vi "GSI-HVSwitch2.get revision.vi"(0 "i ref in":refnum<vi>, 3 "ms timeout (10000)":i32=10000, 5 "error in (no error)":errorcluster) -> (14 "i ref out":refnum<vi>, 15 "revisionType":T1, 16 "revision":string, 17 "timed out":bool, 19 "error out":errorcluster)   [LabVIEW 2014, in "GSI-HVSwitch2.lvlib"]
doc: "Queries the revision number from the device."
uses:
  GSI-HVSwitch2.lvlib
  CSinstr.lib/SDEX/SDEX.revisionType.ctl
  CSCore/CSApplicationBaseClasses/DeviceBase/DeviceBase.lvlib
  CSlibraries-extern/DimLVEvent/NodeMon-LV/LVNodeInfo/LVNodeInfo.lvlib
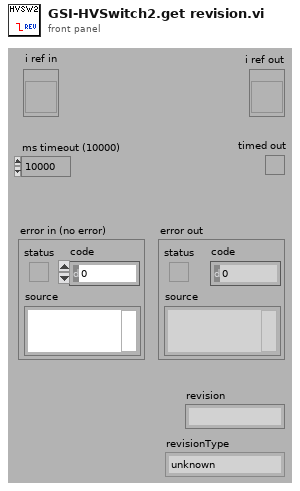
[diagram p1: front panel]
types:
  T1 = typedef "SDEXDriver.lvlib/SDEX.revisionType.ctl" = enum16{"unknown", "hvamp3", "hvswi1", "htrp0", "WDG0"}
  T2 = typedef "GSI-HVSwitch2.lvlib/GSI-HVSwitch2.i attribute.ctl" = cluster{"SDEX VISA Cluster":T3, "SetVoltage SW0":dbl, "SetVoltage SW1":dbl, "ActTempAmp":dbl, "ActTempPS1":dbl, "ActTempPS2":dbl, "mode":T5, "interfaceInitialized":bool, "serviceIDs":cluster{"nomVoltage0ID":i32, "nomVoltage1ID":i32, "actTempAmpID":i32, "actTempPS1ID":i32, "actTempPS2ID":i32, "modeID":i32}, "usedChannels":i32}
  T3 = typedef "SDEXDriver.lvlib/SDEX.VISA Control.ctl" = cluster{"VISA resource name":refnum<visa-resource-name>, "HEX address":u16, "VISA Timeout Value (1000 ms)":u32, "Lock Timeout (1000 ms)":u32, "semaphore":T4, "Baud rate":u32, "revision":T1, "deviceInfo":string}
  T4 = typedef "Semaphore RefNum" = refnum<k1>
  T5 = typedef "GSI-HVSwitch2.lvlib/GSI-HVSwitch2.mode.ctl" = enum16{"unknown", "switch", "stepper"}
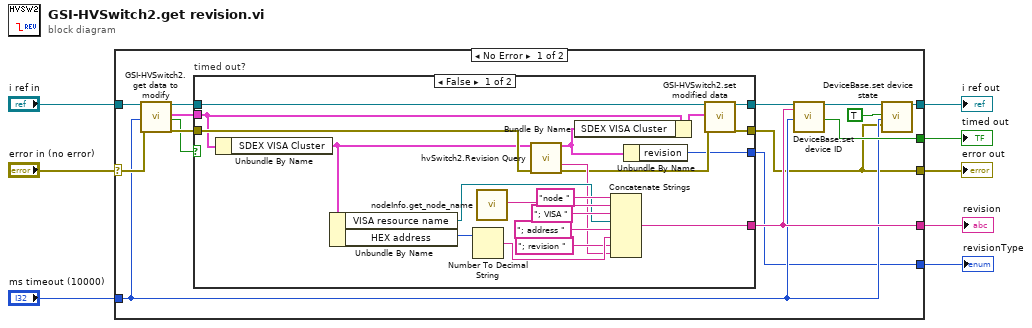
[diagram p0: block diagram]
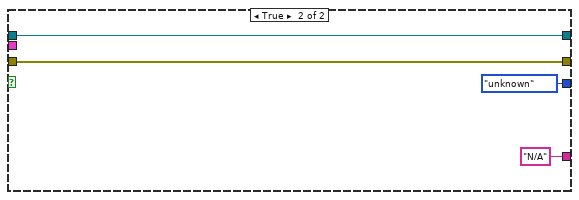
[diagram p2: hidden frame]
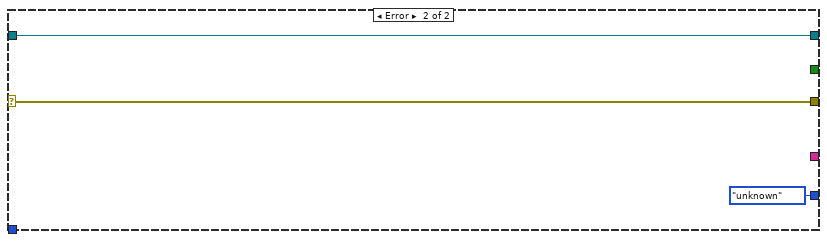
[diagram p3: hidden frame]
diagram:
  n1 = case shown="No Error" "error in (no error)" {
    selector: "error in (no error)" -> [w22 w49]
    tunnel: "i ref in" -> [w23 w50]
    tunnel: "ms timeout (10000)" -> [w12 _]
    tunnel: [w17 w50] -> w6
    tunnel: [w9 w49] -> w5
    tunnel: [w15 _] -> w3
    tunnel: [w19 _] -> w2
    tunnel: [w11 SDEX.revisionType."unknown" ("revision")] -> w1
    frame No Error {
      n2 = call "GSI-HVSwitch2.get data to modify.vi"("i ref in"=w23, "ms timeout (10000)"=w12, "error in (no error)"=w22) -> ("i ref out"=w13:refnum<vi>, "i attribute"=w20:T2, "timed out"=w14:bool, "error out"=w21:errorcluster)  [unwired: 13 in]
      n3 = case "timed out?" shown="False" w14 {
        tunnel: w21 -> [w43 w46]
        tunnel: w20 -> [w28 _]
        tunnel: [w33 "N/A"] -> w15
        tunnel: [w30 w46] -> w9
        tunnel: w13 -> [w32 w47]
        tunnel: [w29 w47] -> w10
        tunnel: [w25 SDEX.revisionType."unknown" ("revision")] -> w11
        frame False {
          n4 = Unbundle By Name(w28) -> ("SDEX VISA Cluster"=w24:T3)
          n5 = Unbundle By Name(w24) -> ("VISA resource name"=w39:refnum<visa-resource-name>, "HEX address"=w37:u16)
          n6 = Number To Decimal String(number=w37) -> (decimal integer string=w36:string)  [unwired: 1 in]
          n7 = call "nodeInfo.get_node_name.vi"() -> ("nodeName"=w41:string)  [unwired: 18 in, 1 out]
          n8 = call "hvSwitch2.Revision Query.vi"("SDEX VISA Cluster"=w24, "error in (no error)"=w43) -> ("dup SDEX VISA Cluster"=w26:T3, "Revision"=w34:string, "error out"=w31:errorcluster)  [unwired: 11 in]
          n9 = Bundle By Name(cluster=w28, "SDEX VISA Cluster"=w26) -> (w27:T2)
          n10 = Concatenate Strings("node " ("string"), w41, "; VISA " ("string"), w39, "; address " ("string"), w36, "; revision " ("string"), w34) -> (w33:string)
          n11 = Unbundle By Name(w26) -> ("revision"=w25:T1)
          n12 = call "GSI-HVSwitch2.set modified data.vi"("i ref in"=w32, "i attribute"=w27, "error in (no error)"=w31) -> ("i ref out"=w29:refnum<vi>, "error out"=w30:errorcluster)  [unwired: 15 in]
        }
        frame True {
        }
      }
      n13 = call "DeviceBase.set device ID.vi"("i ref in"=w10, "deviceID"=w15, "ms timeout (10000)"=w12) -> ("i ref out"=w18:refnum<vi>, "timed out"=w19:bool)  [unwired: 14 in, 1 out]
      n14 = call "DeviceBase.set device state.vi"("i ref in"=w18, "implicit"=TRUE, "ms timeout (10000)"=w12, "device error"=w9) -> ("i ref out"=w17:refnum<vi>)  [unwired: 13 in, 2 out]
    }
    frame Error {
    }
  }
  "error out" <- w5
  "i ref out" <- w6
  "timed out" <- w2
  "revision" <- w3
  "revisionType" <- w1
